vi "MovingAverageFilter.vi"(7 "half-width":i32=2, 11 "X":dbl[](array[numeric])) -> (3 "Filtered X":dbl[](array[numeric]))   [LabVIEW 2022 SP3]
uses:
  <vilib>/Analysis/3filter.llb/Zero Phase Filter (DBL).vi
  <vilib>/Analysis/NI_AALBase.lvlib
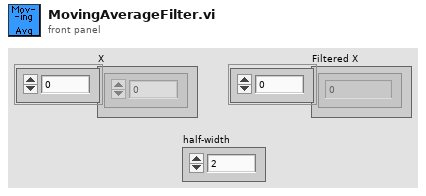
[diagram p1: front panel]
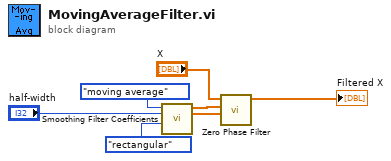
[diagram p0: block diagram]
diagram:
  n1 = call <vilib>:"Smoothing Filter Coefficients.vi"("shape"=enum16{"rectangular", "triangular"}."rectangular", "half-width"="half-width", "type"=enum16{"moving average", "exponential"}."moving average") -> ("forward coefficients"=w5:dbl[], "reverse coefficients"=w4:dbl[])  [unwired: 6 in, 1 out]
  n2 = call-poly <vilib>:"Zero Phase Filter.vi"("Forward Coefficients"=w5, "Reverse Coefficients"=w4, "X"="X") -> ("Filtered X"=→"Filtered X":dbl[])  [unwired: 7 in, 1 out]
